vi "Ex2 gripper.vi"() -> ()   [LabVIEW 2013]
uses:
  ROS/Code/SubVIs/BaxterSide.ctl
panel:
  in  "Pause":u32=5000
  out "Status":string
  in  "Side":T1=enum."right"
  # "Hit run to close and open the gripper"
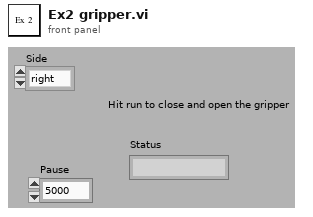
[diagram p1: front panel]
types:
  T1 = typedef "BaxterSide.ctl" = enum16{"left", "right"}
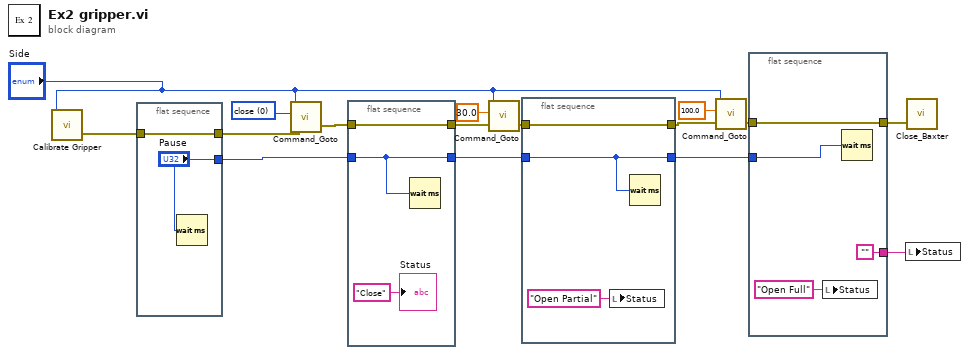
[diagram p0: block diagram]
diagram:
  w16 = u16 0 items=["close"=0, "open"=100] ("left gripper")
  n1 = call "Calibrate Gripper.vi"("Side"="Side") -> ("error out"=w2:errorcluster)  [unwired: 5 in]
  n2 = flat-sequence {
    tunnel: ["Pause"] -> w5
    tunnel: w2 -> [w18]
    tunnel: [w18] -> w1
    frame #0 {
      n3 = Wait (ms)(milliseconds to wait="Pause") -> ()  [unwired: 1 out]
    }
  }
  n4 = call "Command_Goto.vi"("Side"="Side", "Desired Position"=w16, "error in"=w1) -> ("error out"=w14:errorcluster)  [unwired: 3 in]
  n5 = flat-sequence {
    tunnel: [w21] -> w15
    tunnel: w14 -> [w21]
    tunnel: w5 -> [w19]
    tunnel: [w19] -> w4
    frame #0 {
      n6 = Wait (ms)(milliseconds to wait=w19) -> ()  [unwired: 1 out]
      "Status" <- "Close" ("Status")
    }
  }
  n7 = call "Command_Goto.vi"("Side"="Side", "Desired Position"=sgl 30.0, "error in"=w15) -> ("error out"=w12:errorcluster)  [unwired: 3 in]
  n8 = flat-sequence {
    tunnel: [w24] -> w9
    tunnel: w12 -> [w24]
    tunnel: w4 -> [w22]
    tunnel: [w22] -> w3
    frame #0 {
      n9 = local write "Status"("Open Partial" ("Status")) -> ()
      n10 = Wait (ms)(milliseconds to wait=w22) -> ()  [unwired: 1 out]
    }
  }
  n11 = call "Command_Goto.vi"("Side"="Side", "Desired Position"=sgl 100.0, "error in"=w9) -> ("error out"=w11:errorcluster)  [unwired: 3 in]
  n12 = flat-sequence {
    tunnel: [w28] -> w8
    tunnel: w11 -> [w28]
    tunnel: [""] -> w6
    tunnel: w3 -> [w25]
    frame #0 {
      n13 = local write "Status"("Open Full" ("Status")) -> ()
      n14 = Wait (ms)(milliseconds to wait=w25) -> ()  [unwired: 1 out]
    }
  }
  n15 = local write "Status"(w6) -> ()
  n16 = call "Close_Baxter.vi"("error in"=w8) -> ()  [unwired: 3 in, 1 out]
